vi "express_TDMS.vi"() -> ()   [LabVIEW 2018]
panel:
  out "웨이브폼 그래프":dynamicdata(graph)
  in  "정지 버튼":bool
  out "웨이브폼 차트":dbl(graph)
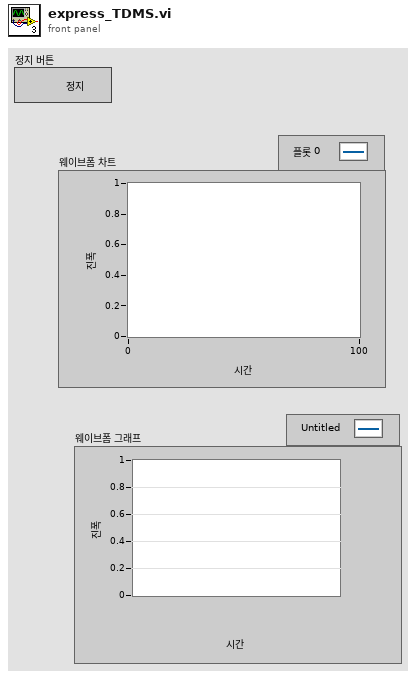
[diagram p1: front panel]
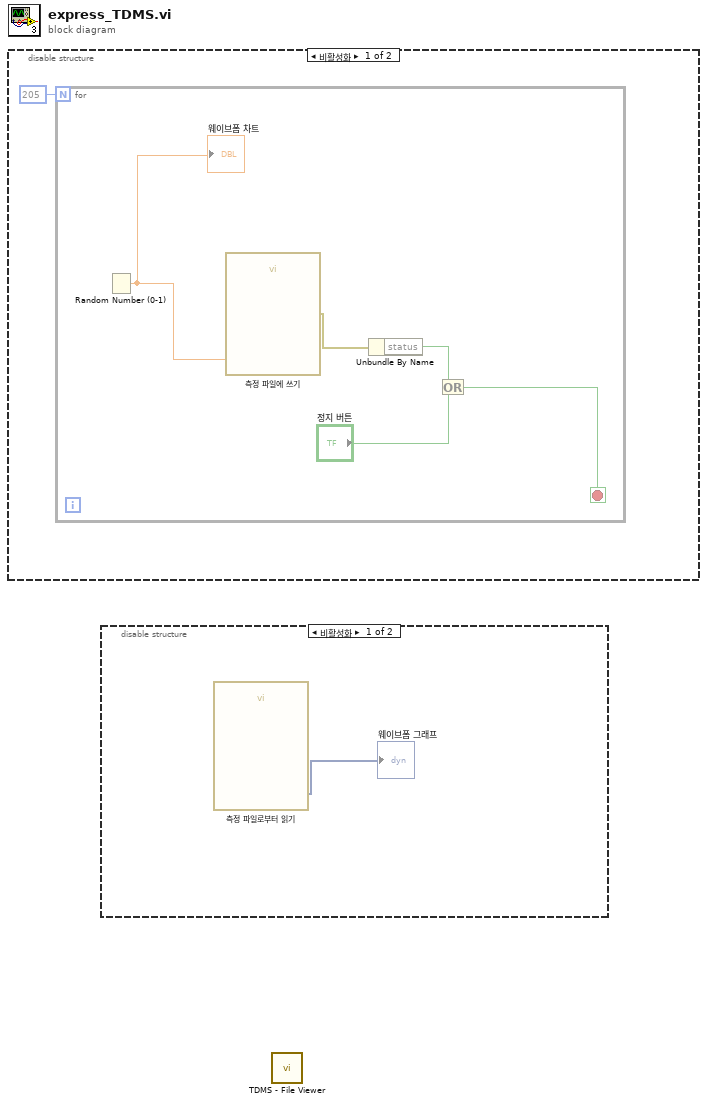
[diagram p0: block diagram]
diagram:
  n1 = disable-structure shown="비활성화" {
    frame Disabled {
      n2 = for {
        N: 205 -> [_]
        stop <- w2 stop-if-true
        n3 = Random Number (0-1)() -> (number: 0 to 1=w6:dbl)
        "웨이브폼 차트" <- w6
        n4 = call "측정 파일에 쓰기"("Signals"=w6) -> ("error out"=w4:errorcluster)  [unwired: 16 in, 2 out]
        n5 = Unbundle By Name(w4) -> ("status"=w3:bool)
        n6 = Or(x=w3, y="정지 버튼") -> (x .or. y?=w2:bool)
      }
    }
    frame Enabled {
    }
  }
  n7 = disable-structure shown="비활성화" {
    frame Disabled {
      n8 = call "측정 파일로부터 읽기"() -> ("Signals"=→"웨이브폼 그래프":dynamicdata)  [unwired: 6 in, 5 out]
    }
    frame Enabled {
    }
  }
  n9 = call <vilib>:"TDMS - File Viewer.vi"() -> ()  [unwired: 6 in, 2 out]
